vi "Population Recombination.vi"(6 "Mutation Rate":dbl, 7 "Population Size":i32, 8 "error in":errorcluster, 9 "Recombination Type":enum16{"Gene Coin Flip", "Pivot Crossover"}(ring), 10 "Parent Pool Behavior":T1(ring), 11 "Parent Chromosome Pool In":refnum<class "IChromosome.lvclass">[](array[class])) -> (0 "error out":errorcluster, 3 "Children Chromosomes Out":refnum<class "IChromosome.lvclass">[](array[class]))   [LabVIEW 2016, in "IPopulation.lvclass"]
uses:
  IPopulation.lvclass
  IChromosome/IChromosome.lvclass
  IChromosome/IChromosome.lvclass/IChromosome.ctl
  <userlib>/_OpenG.lib/numeric/numeric.llb/Random Number Within Range - I32__ogtk.vi
  IGene/IGene.lvclass
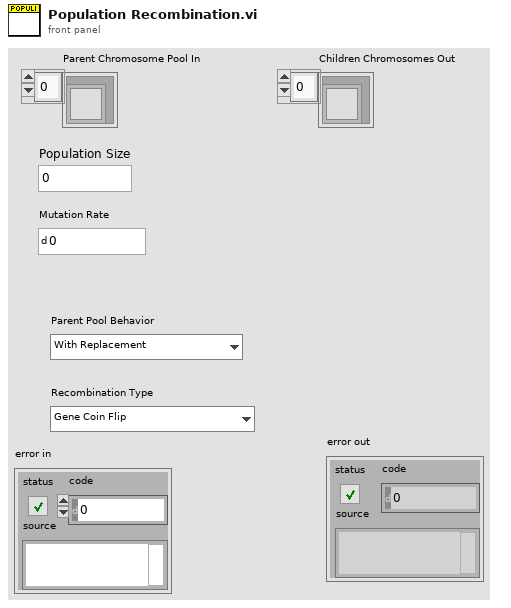
[diagram p1: front panel]
types:
  T1 = enum16{"With Replacement", "Without Replacement"}
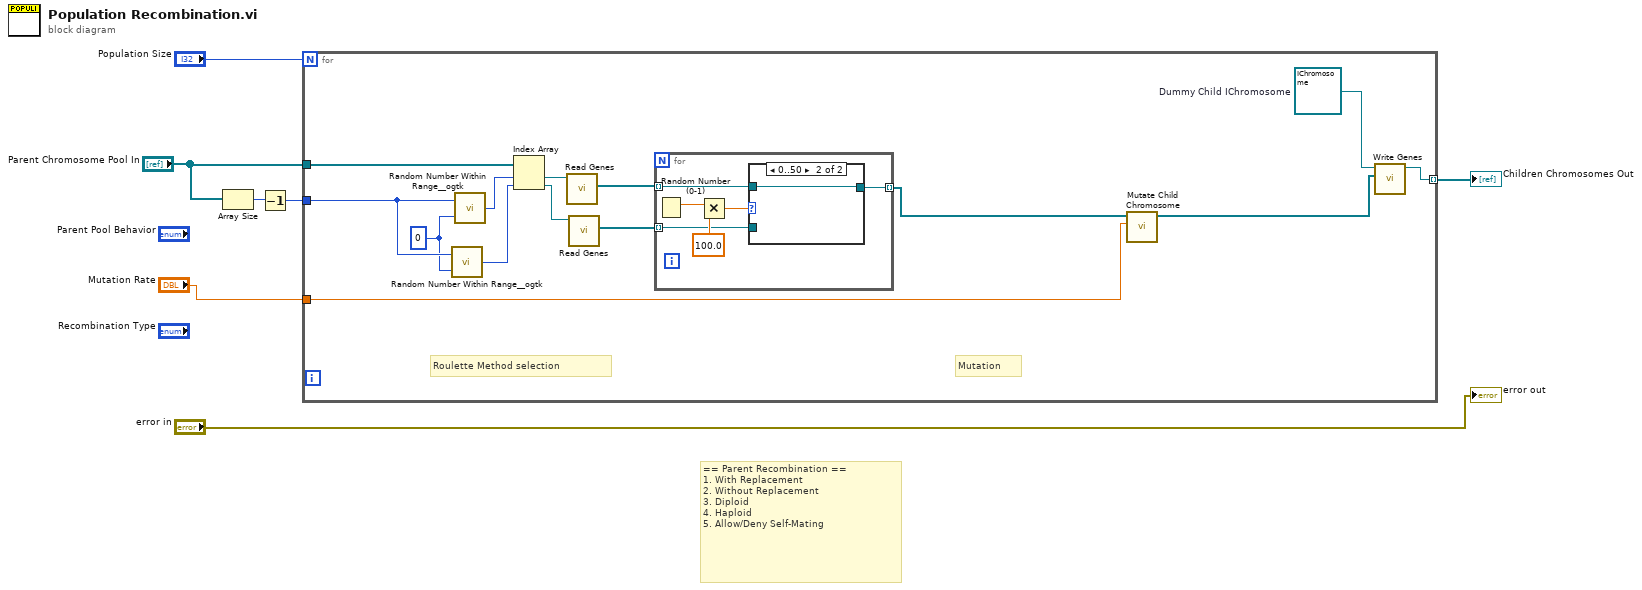
[diagram p0: block diagram]
diagram:
  # "== Parent Recombination ==\n1. With Replacement\n2. Without Replacement\n3. Diploid\n4. Haploid\n5. Allow/Deny Self-Mating"
  n1 = Array Size(array="Parent Chromosome Pool In") -> (size(s)=w7:i32)
  n2 = Decrement(x=w7) -> (x-1=w5:i32)
  n3 = for {
    N: "Population Size" -> [_]
    tunnel: w5 -> [w21]
    tunnel: "Parent Chromosome Pool In" -> [w11]
    tunnel: [w16] -> w6 mode=indexing
    tunnel: "Mutation Rate" -> [w8]
    w9 = refnum<class "IChromosome.lvclass"> refnum  # Dummy Child IChromosome
    w15 = 0 ("Low")
    # "Roulette Method selection"
    # "Mutation"
    n4 = call-poly <userlib>:"Random Number Within Range__ogtk.vi"("High"=w21, "Low"=w15) -> ("Random Number"=w20:i32)  [unwired: 3 in]
    n5 = call-poly <userlib>:"Random Number Within Range__ogtk.vi"("High"=w21, "Low"=w15) -> ("Random Number"=w14:i32)  [unwired: 3 in]
    n6 = Index Array(array=w11, index #1=w14, index #2=w20) -> (element #1=w10:refnum<class "IChromosome.lvclass">, element #2=w19:refnum<class "IChromosome.lvclass">)
    n7 = call "Read Genes.vi"("IChromosome in"=w10) -> ("Genes"=w18:refnum<class "IGene.lvclass">[])  [unwired: 8 in, 2 out]
    n8 = call "Read Genes.vi"("IChromosome in"=w19) -> ("Genes"=w17:refnum<class "IGene.lvclass">[])  [unwired: 8 in, 2 out]
    n9 = for {
      tunnel: w18 -> [w24] mode=indexing
      tunnel: w17 -> [w23] mode=indexing
      tunnel: [w22] -> w13 mode=indexing
      n10 = Random Number (0-1)() -> (number: 0 to 1=w27:dbl)
      n11 = Multiply(x=w27, y=100.0) -> (x*y=w25:dbl)
      n12 = case shown="0..50" w25 {
        tunnel: w24 -> [_ w29]
        tunnel: w23 -> [w28 _]
        tunnel: [w28 w29] -> w22
        frame 51.., Default {
        }
        frame 0..50 {
        }
      }
    }
    n13 = call "Mutate Child Chromosome.vi"("Mutation Rate"=w8, "Child Chromosome In"=w13) -> ("Child Chromosome out"=w12:refnum<class "IGene.lvclass">[])  [unwired: 9 in]
    n14 = call "Write Genes.vi"("Genes"=w12, "IChromosome in"=w9) -> ("IChromosome out"=w16:refnum<class "IChromosome.lvclass">)  [unwired: 8 in, 1 out]
  }
  "Children Chromosomes Out" <- w6
  "error out" <- "error in"
